vi "TrajectoryUtil_MakeWeightedWayPoint.vi"(8 "Weight":dbl, 9 "Travel Angle Radians":dbl, 10 "Y_M":dbl, 11 "X_M":dbl) -> (3 "WEIGHTED_WAYPOINT":T1={"TRANSLATION"={"X"=0.0, "Y"=0.0}, "ROTATION"={"VALUE"=0.0, "COS"=1.0, "SIN"=0.0}, "SCALAR"=0.0} {"SCALAR" format="%14.3f"; "ROTATION"."SIN" format="%13.4f"; "ROTATION"."COS" format="%13.4f"; "ROTATION"."VALUE" format="%13.4f"; "TRANSLATION"."Y" format="%14.3f"; "TRANSLATION"."X" format="%14.3f"})   [LabVIEW 2019, in "Trajectory_Library.lvlib"]
doc: "Creates a waypoint data structure from individual inputs. \n\nInputs are all SI units (Meters, Radians)"
uses:
  Trajectory_Library.lvlib
  WEIGHTED_WAYPOINT.ctl
  TRANSLATION2D.ctl
  ROTATION2D.ctl
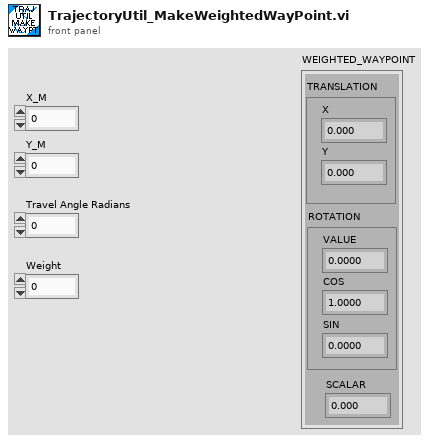
[diagram p1: front panel]
types:
  T1 = typedef "Trajectory_Library.lvlib/WEIGHTED_WAYPOINT.ctl" = cluster{"TRANSLATION":T2, "ROTATION":T3, "SCALAR":dbl}
  T2 = typedef "Trajectory_Library.lvlib/TRANSLATION2D.ctl" = cluster{"X":dbl, "Y":dbl}
  T3 = typedef "Trajectory_Library.lvlib/ROTATION2D.ctl" = cluster{"VALUE":dbl, "COS":dbl, "SIN":dbl}
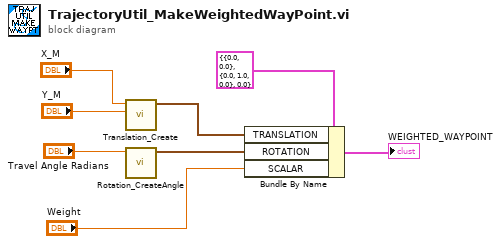
[diagram p0: block diagram]
diagram:
  n1 = call "Translation_Create.vi"("Y"="Y_M", "X"="X_M") -> ("TRANSLATION"=w6:T2)  [unwired: 9 in]
  n2 = call "Rotation_CreateAngle.vi"("Angle"="Travel Angle Radians") -> ("ROTATION"=w5:T3)  [unwired: 10 in]
  n3 = Bundle By Name(cluster=T1 {"TRANSLATION"={"X"=0.0, "Y"=0.0}, "ROTATION"={"VALUE"=0.0, "COS"=1.0, "SIN"=0.0}, "SCALAR"=0.0} ("WEIGHTED_WAYPOINT"), "TRANSLATION"=w6, "ROTATION"=w5, "SCALAR"="Weight") -> (→"WEIGHTED_WAYPOINT":T1)
